vi "acquisitionFindFrameInBuffer.vi"(2 "startBufferIndex":i32, 3 "frameCounts":i32[](array[numeric]), 4 "hamamatsuFrameAvailableReferences":refnum<data-value>[](array[refnum])) -> (0 "success":bool, 1 "frameIndices":i32[](array[numeric]))   [LabVIEW 2017]
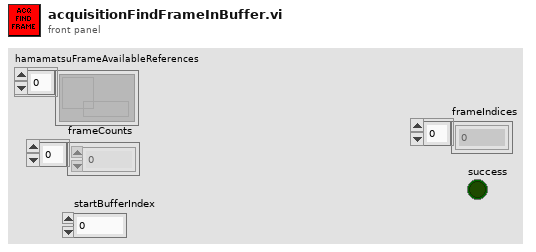
[diagram p1: front panel]
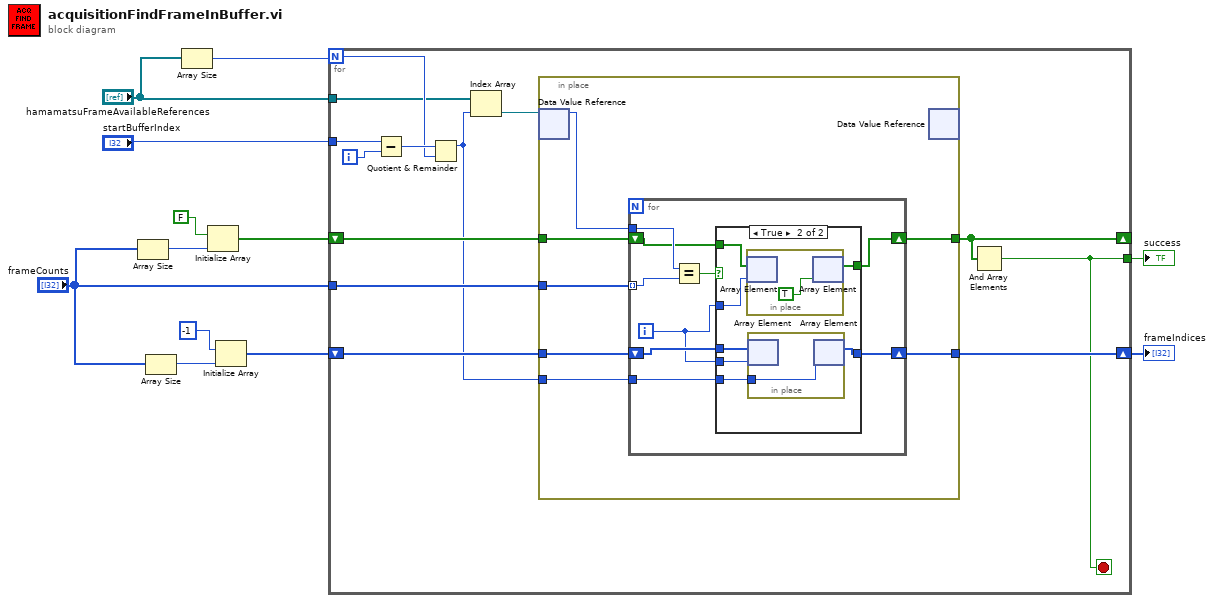
[diagram p0: block diagram]
diagram:
  n1 = Array Size(array="frameCounts") -> (size(s)=w9:i32)
  n2 = Array Size(array="frameCounts") -> (size(s)=w6:i32)
  n3 = Array Size(array="hamamatsuFrameAvailableReferences") -> (size(s)=w12:i32)
  n4 = Initialize Array(FALSE, w9) -> (w7:bool[])
  n5 = Initialize Array(-1, w6) -> (w3:i32[])
  n6 = for {
    N: w12 -> [w22]
    tunnel: "startBufferIndex" -> [w25]
    tunnel: "hamamatsuFrameAvailableReferences" -> [w21]
    tunnel: "frameCounts" -> [w19]
    shift-right: [w14] -> _
    shift-left: w7 -> [w18]
    shift-right: [w15] -> w1
    shift-left: w3 -> [w17]
    tunnel: [w13] -> w2
    i -> [w24]
    stop <- w13 stop-if-true
    n7 = Subtract(x=w25, y=w24) -> (x-y=w23:i32)
    n8 = Quotient & Remainder(x=w23, y=w22) -> (x-y*floor(x/y)=w16:i32)  [unwired: 1 out]
    n9 = Index Array(array=w21, index=w16) -> (element=w20:refnum<data-value>)
    n10 = in-place {
      in-place-border: w19 -> [w32]
      in-place-border: w18 -> [w31]
      in-place-border: w17 -> [w29]
      in-place-border: w16 -> [w28]
      in-place-border: [w27] -> w14
      in-place-border: [w26] -> w15
      n11 = in-place-dvr #1(w20) -> (w30:i32)  [unwired: 1 out]
      n12 = for {
        tunnel: w32 -> [w40] mode=indexing
        tunnel: w30 -> [w41]
        shift-right: [w37] -> w27
        shift-left: w31 -> [w38]
        shift-right: [w33] -> w26
        shift-left: w29 -> [w36]
        tunnel: w28 -> [w34]
        i -> [w35]
        n13 = Equal?(x=w41, y=w40) -> (x = y?=w39:bool)
        n14 = case shown="True" w39 {
          tunnel: w38 -> [w43 w50]
          tunnel: w35 -> [_ w49]
          tunnel: [w43 w48] -> w37
          tunnel: w36 -> [w42 w47]
          tunnel: w35 -> [_ w46]
          tunnel: w34 -> [_ w45]
          tunnel: [w42 w44] -> w33
          frame False {
          }
          frame True {
            n15 = in-place {
              n16 = in-place-array #2(w50, w49) -> ()  [unwired: 1 out]
              n17 = in-place-array #2(TRUE) -> (w48:bool[])  [unwired: 1 out]
            }
            n18 = in-place {
              in-place-border: w45 -> [w51]
              n19 = in-place-array #3(w47, w46) -> ()  [unwired: 1 out]
              n20 = in-place-array #3(w51) -> (w44:i32[])  [unwired: 1 out]
            }
          }
        }
      }
      n21 = in-place-dvr #1() -> ()  [unwired: 1 in, 2 out]
    }
    n22 = And Array Elements(Boolean array=w14) -> (logical AND=w13:bool)
  }
  "success" <- w2
  "frameIndices" <- w1
